vi "EL-RIO-CM v1.0 Configure Encoder.vi"(8 "error in (no error)":errorcluster, 9 "Encoder Configuration v1.0":T1, 10 "Encoder Channel":T3, 11 "myRIO Ref In":T4) -> (0 "error out":errorcluster)   [LabVIEW 2021]
uses:
  <vilib>/myRIO/Common/Instrument Driver Framework/Utilities/typedefs/myRIO v1.0 Reference.ctl
  <vilib>/myRIO/Common/Instrument Driver Framework/Utilities/typedefs/Generic FPGA Reference.ctl
  <vilib>/myRIO/Common/Instrument Driver Framework/myRIO v1.0/Encoder/typedefs/Encoder Channels Enum.ctl
  <vilib>/myRIO/Common/Instrument Driver Framework/myRIO v1.0/Encoder/typedefs/Encoder Configuration v1.0.ctl
  <vilib>/myRIO/Common/Instrument Driver Framework/myRIO v1.0/Encoder/typedefs/Encoder Signal Mode.ctl
  <vilib>/myRIO/Common/Instrument Driver Framework/myRIO v1.0/Encoder/typedefs/Encoder Config Manager Action Enum.ctl
  <vilib>/myRIO/Common/Instrument Driver Framework/myRIO v1.0/Encoder/typedefs/Encoder Channels FPGA Reference.ctl
  <vilib>/rvi/errors/niLvFpgaAdjustHostInterfaceError.vi
  <vilib>/rvi/interface/nirviReadWriteControl/nirviReadWriteControl.xnode
  <vilib>/rvi/interface/Simulation/niFpgaSimulationCallBeginRW.vi
  NiFpgaLv.dll
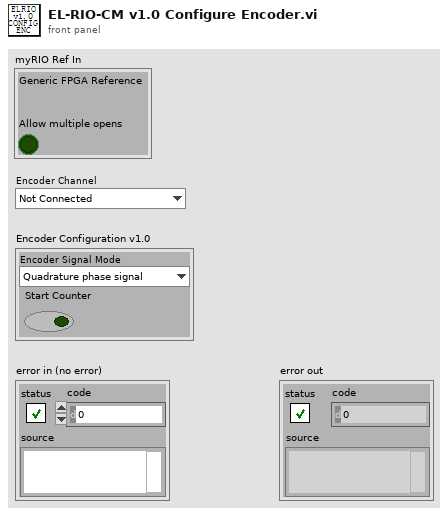
[diagram p1: front panel]
types:
  T1 = typedef "Encoder Configuration v1.0.ctl" = cluster{"Encoder Signal Mode":T2, "Start Counter":bool}
  T2 = typedef "Encoder Signal Mode.ctl" = enum16{"Quadrature phase signal", "Step and direction signal"}
  T3 = typedef "Encoder Channels Enum.ctl" = enum16{"Not Connected", "C/ENC0", "C/ENC1", "A/ENC", "A/ENC0", "A/ENC1", "A/ENC2", "A/ENC3", "A/ENC4", "A/ENC5", "A/ENC6", "A/ENC7", "A/ENC8", "A/ENC9", "B/ENC", "B/ENC0", "B/ENC1", "B/ENC2", "B/ENC3", "B/ENC4", "B/ENC5", "B/ENC6", "B/ENC7", "B/ENC8", "B/ENC9", "DIO/ENC0", "DIO/ENC1", "DIO/ENC2", "DIO/ENC3", "DIO/ENC4"}
  T4 = typedef "myRIO v1.0 Reference.ctl" = cluster{"Generic FPGA Reference":T5, "Allow multiple opens":bool}
  T5 = typedef "Generic FPGA Reference.ctl" = refnum<k20>
  T6 = typedef "Encoder Config Manager Action Enum.ctl" = enum16{"Do Nothing", "Store", "Clear"}
  T7 = typedef "Encoder Channels FPGA Reference.ctl" = refnum<k20>
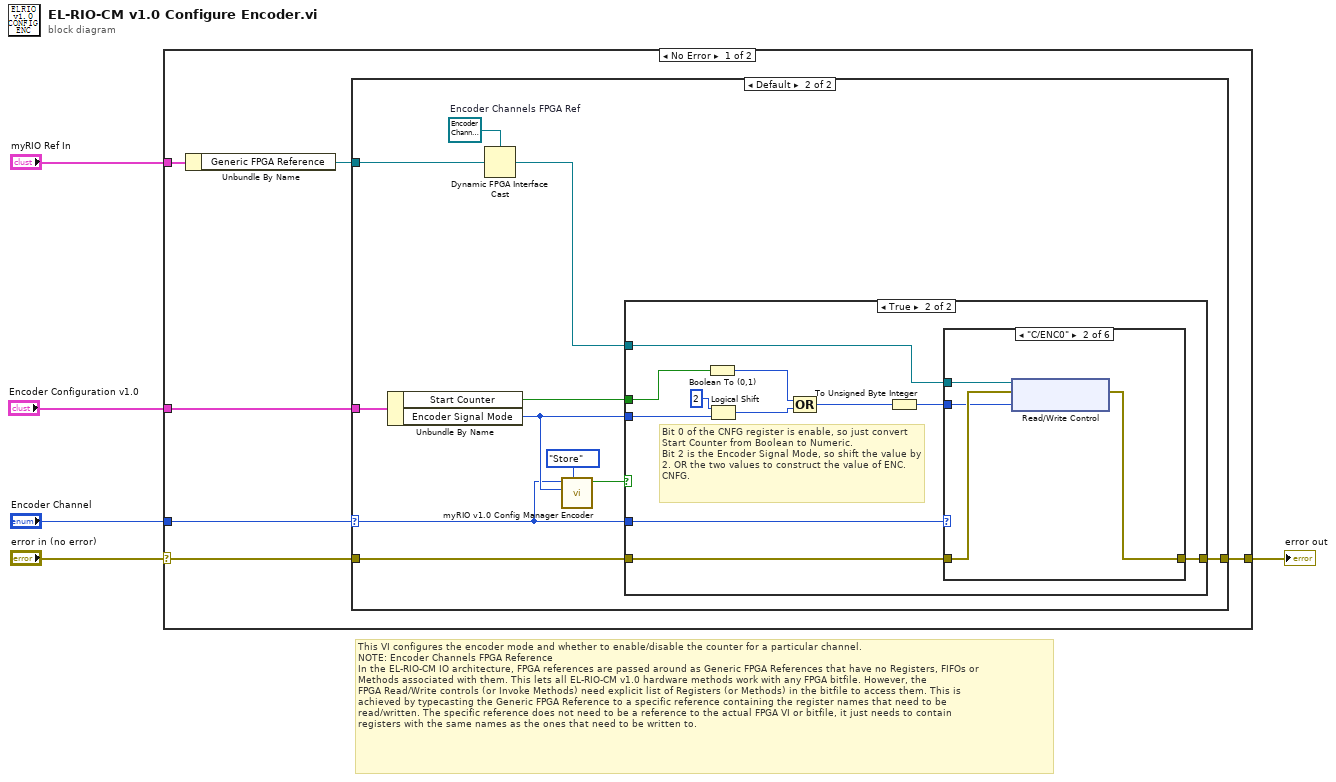
[diagram p0: block diagram]
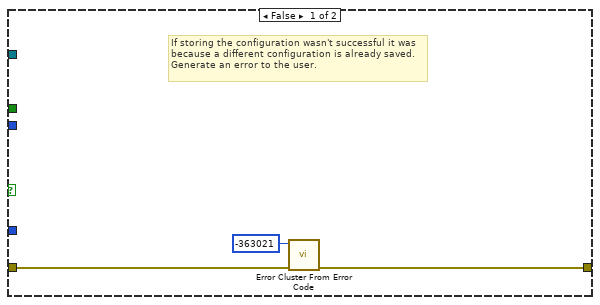
[diagram p3: hidden frame]
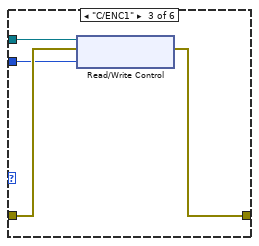
[diagram p5: hidden frame]
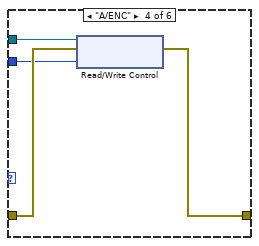
[diagram p6: hidden frame]
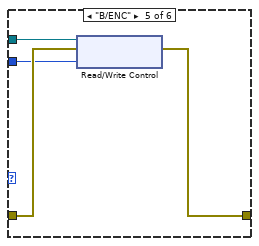
[diagram p7: hidden frame]
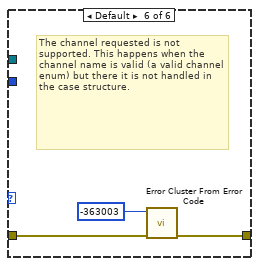
[diagram p8: hidden frame]
diagram:
  # "This VI configures the encoder mode and whether to enable/disable the counter for a particular channel.\nNOTE: Encoder Channels FPGA Reference\nIn the EL-RIO-CM IO architecture, FPGA references are passed around as Generic FPGA References that have no Registers, FIFOs or\nMethods associated with them. This lets all EL-RIO-CM v1.0 hardware methods work with any FPGA bitfile. However, the \nFPGA Read/Write controls (or Invoke Methods) need explicit list of Registers (or Methods) in the bitfile to access them. This is \nachieved by typecasting the Generic FPGA Reference to a specific reference containing the register names that need to be \nread/written. The specific reference does not need to be a reference to the actual FPGA VI or bitfile, it just needs to contain \nregisters with the same names as the ones that need to be written to."
  n1 = case shown="No Error" "error in (no error)" {
    selector: "error in (no error)" -> [w10 w58]
    tunnel: [w11 w58] -> w5
    tunnel: "myRIO Ref In" -> [w9 _]
    tunnel: "Encoder Channel" -> [w8 _]
    tunnel: "Encoder Configuration v1.0" -> [w7 _]
    frame No Error {
      n2 = Unbundle By Name(w9) -> ("Generic FPGA Reference"=w6:T5)
      n3 = case shown="Default" w8 {
        selector: w8 -> [_ w14]
        tunnel: [w12 w21] -> w11
        tunnel: w10 -> [w12 w20]
        tunnel: w6 -> [_ w19]
        tunnel: w7 -> [_ w18]
        frame "Not Connected" {
        }
        frame Default {
          w23 = T7 refnum  # Encoder Channels FPGA Ref
          n4 = Unbundle By Name(w18) -> ("Start Counter"=w17:bool, "Encoder Signal Mode"=w15:T2)
          n5 = Dynamic FPGA Interface Cast(Session In=w23, Type=w19) -> (Session Out=w22:T7)
          n6 = call <vilib>:"myRIO v1.0 Config Manager Encoder.vi"("Action"=Encoder_Config_Manager_Action_Enum."Store", "Encoder Signal Mode"=w15, "Encoder Channel"=w14) -> ("Success?"=w13:bool)  [unwired: 8 in]
          n7 = case shown="True" w13 {
            tunnel: w22 -> [_ w37]
            tunnel: [w25 w36] -> w21
            tunnel: w20 -> [w26 w35]
            tunnel: w17 -> [_ w32]
            tunnel: w15 -> [_ w28]
            tunnel: w14 -> [_ w27]
            frame False {
              # "If storing the configuration wasn't successful it was because a different configuration is already saved. Generate an error to the user."
              n8 = call <vilib>:"Error Cluster From Error Code.vi"("error in (no error)"=w26, "error code (0)"=-363021) -> ("error out"=w25:errorcluster)  [unwired: 7 in]
            }
            frame True {
              # "Bit 0 of the CNFG register is enable, so just convert Start Counter from Boolean to Numeric.\nBit 2 is the Encoder Signal Mode, so shift the value by 2. OR the two values to construct the value of ENC.CNFG."
              n9 = Boolean To (0,1)(Boolean=w32) -> (0, 1=w31:i16)
              n10 = Logical Shift(y=i8 2, x=w28) -> (x << y=w29:u32)
              n11 = Compound Arithmetic op=OR(w31, w29) -> (w30:u32)
              n12 = To Unsigned Byte Integer(number=w30) -> (unsigned 8bit integer=w33:u8)
              n13 = case shown="\"C/ENC0\"" w27 {
                tunnel: w35 -> [w38 w41 w45 w49 w53 w55]
                tunnel: [w38 w39 w43 w47 w51 w56] -> w36
                tunnel: w37 -> [_ w42 w46 w50 w54 _]
                tunnel: w33 -> [_ w40 w44 w48 w52 _]
                frame "Not Connected" {
                }
                frame "C/ENC0" {
                  n14 = xnode "Read/Write Control"("FPGA VI Reference In"=w42, "error in"=w41, "ENC.C_0.CNFG"=w40) -> ("error out"=w39:errorcluster)  [unwired: 1 out]
                }
                frame "C/ENC1" {
                  n15 = xnode "Read/Write Control"("FPGA VI Reference In"=w46, "error in"=w45, "ENC.C_1.CNFG"=w44) -> ("error out"=w43:errorcluster)  [unwired: 1 out]
                }
                frame "A/ENC" {
                  n16 = xnode "Read/Write Control"("FPGA VI Reference In"=w50, "error in"=w49, "ENC.A.CNFG"=w48) -> ("error out"=w47:errorcluster)  [unwired: 1 out]
                }
                frame "B/ENC" {
                  n17 = xnode "Read/Write Control"("FPGA VI Reference In"=w54, "error in"=w53, "ENC.B.CNFG"=w52) -> ("error out"=w51:errorcluster)  [unwired: 1 out]
                }
                frame Default {
                  # "The channel requested is not supported. This happens when the channel name is valid (a valid channel enum) but there it is not handled in the case structure."
                  n18 = call <vilib>:"Error Cluster From Error Code.vi"("error in (no error)"=w55, "error code (0)"=-363003) -> ("error out"=w56:errorcluster)  [unwired: 7 in]
                }
              }
            }
          }
        }
      }
    }
    frame Error {
      # "There is an incoming error so there is nothing to do."
    }
  }
  "error out" <- w5
